vi "Highlight Text.vi"(7 "Values":refnum<vi>, 8 "error in (no error)":errorcluster, 9 "ASCII":refnum<vi>, 10 "Hex":refnum<vi>, 11 "queue data in":T1={"server ID"=refnum, "Buffer data"={"decimation"=0, "avg bandwidth"=0.0, "channels"=[], "byte order"=enum."little-endian", "buffer descriptor"={"buffer type"=enum."Engine", "plugin id"=0, "group id"=0, "transfer id"=0, "offset"=0, "length"=0}, "values channels"={"index"=0, "count"=0, "engine offset"=0}, "select start offset"=18446744073709551615, "select end offset"=0, "channel index"=-1}} {"Buffer data"."channels"."configuration"."string offset" format="%d bytes"; "Buffer data"."avg bandwidth" format="%.0g bytes"}) -> (0 "error out":errorcluster, 3 "queue data out":T1={"server ID"=refnum, "Buffer data"={"decimation"=0, "avg bandwidth"=0.0, "channels"=[], "byte order"=enum."little-endian", "buffer descriptor"={"buffer type"=enum."Engine", "plugin id"=0, "group id"=0, "transfer id"=0, "offset"=0, "length"=0}, "values channels"={"index"=0, "count"=0, "engine offset"=0}, "select start offset"=18446744073709551615, "select end offset"=0, "channel index"=-1}} {"Buffer data"."channels"."configuration"."string offset" format="%d bytes"; "Buffer data"."avg bandwidth" format="%.0g bytes"})   [LabVIEW 2017, in "DSF Core.lvlib"]
uses:
  DSF Core.lvlib
  Buffer Reader/Queue Data.ctl
  Buffer Reader/Buffer Data.ctl
  Classes/Configuration/Core/Transfer/Channel Configuration.ctl
  Typedefs/Core Channel Configuration.ctl
  Typedefs/DSF Data Type.ctl
  Typedefs/DSF Settings Info.ctl
  Typedefs/DSF Byte Order.ctl
  Classes/Thread/Data Server/DSF Buffer Subset Descriptor.ctl
  Typedefs/DSF Buffer Type.ctl
  Values Channels.ctl
  Classes/Configuration/Core/Channel/Channel Configuration.lvclass
  Classes/Configuration/Core/Transfer/Transfer Configuration.lvclass
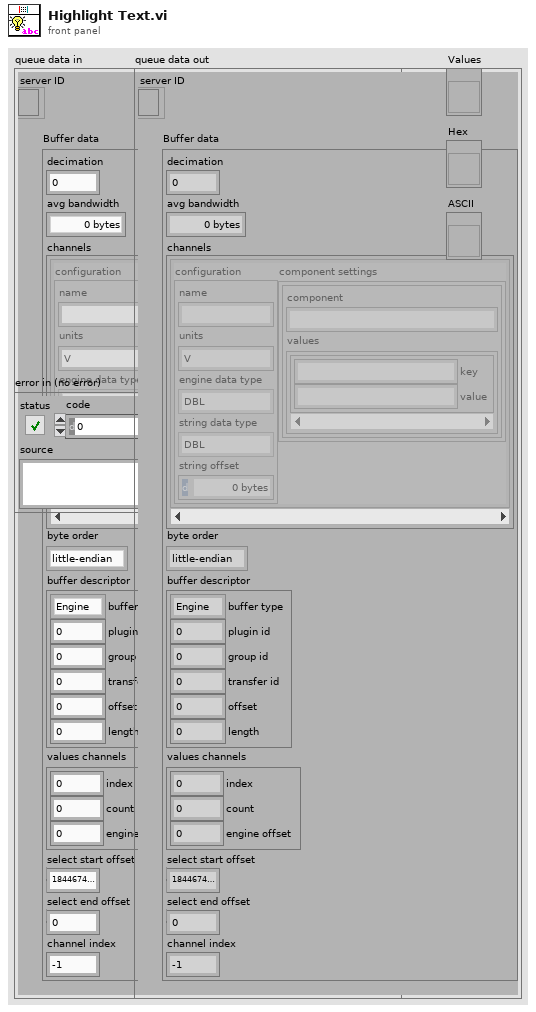
[diagram p1: front panel]
types:
  T1 = typedef "DSF Core.lvlib/Queue Data.ctl" = cluster{"server ID":refnum<k5>, "Buffer data":T2}
  T2 = typedef "DSF Core.lvlib/Buffer Data.ctl" = cluster{"decimation":u64, "avg bandwidth":dbl, "channels":T3[], "byte order":T7, "buffer descriptor":T8, "values channels":T10, "select start offset":u64, "select end offset":u64, "channel index":i32}
  T3 = typedef "DSF Core.lvlib/Transfer Configuration.lvclass/Channel Configuration.ctl" = cluster{"configuration":T4, "component settings":T6[]}
  T4 = typedef "DSF Core.lvlib/Channel Configuration.lvclass/Core Channel Configuration.ctl" = cluster{"name":string, "units":string, "engine data type":T5, "string data type":T5, "string offset":u64}
  T5 = typedef "DSF Core.lvlib/DSF Data Type.ctl" = enum8{"Bool", "SGL", "DBL", "I8", "I16", "I32", "I64", "U8", "U16", "U32", "U64"}
  T6 = typedef "DSF Core.lvlib/DSF Settings Info.ctl" = cluster{"component":string, "values":cluster{"key":string, "value":string}[]}
  T7 = typedef "DSF Core.lvlib/DSF Byte Order.ctl" = enum8{"big-endian", "little-endian"}
  T8 = typedef "DSF Core.lvlib/DSF Buffer Subset Descriptor.ctl" = cluster{"buffer type":T9, "plugin id":i32, "group id":i32, "transfer id":i32, "offset":u64, "length":i64}
  T9 = typedef "DSF Core.lvlib/DSF Buffer Type.ctl" = enum16{"Engine", "String"}
  T10 = typedef "DSF Core.lvlib/Values Channels.ctl" = cluster{"index":i32, "count":i32, "engine offset":u64}
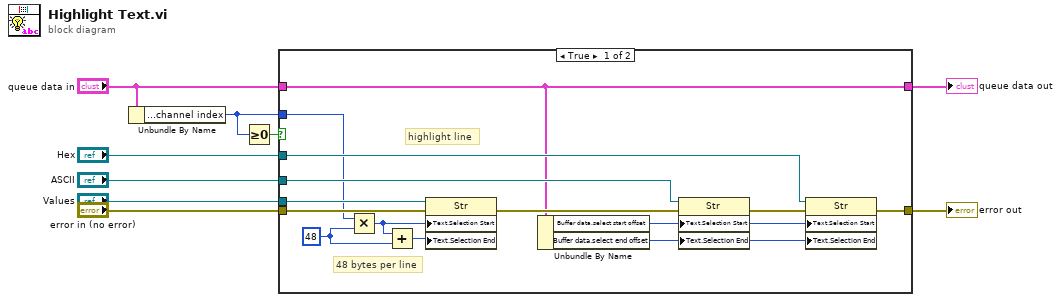
[diagram p0: block diagram]
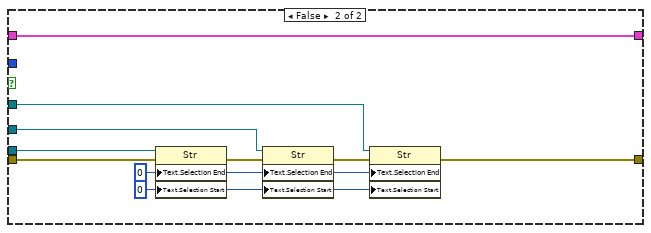
[diagram p2: hidden frame]
diagram:
  n1 = Unbundle By Name("queue data in") -> ("Buffer data.channel index"=w1:i32)
  n2 = Greater Or Equal To 0?(x=w1) -> (x >= 0?=w5:bool)
  n3 = case shown="True" w5 {
    tunnel: "ASCII" -> [w19 w28]
    tunnel: "Hex" -> [w14 w29]
    tunnel: [w12 w32] -> w9
    tunnel: "queue data in" -> [w11 w26]
    tunnel: [w11 w26] -> w8
    tunnel: "error in (no error)" -> [w22 w31]
    tunnel: "Values" -> [w20 w30]
    tunnel: w1 -> [w10 _]
    frame True {
      w17 = 48 ("y")
      # "highlight line"
      # "48 bytes per line"
      n4 = Multiply(x=w10, y=w17) -> (x*y=w15:i32)
      n5 = Add(x=w15, y=w17) -> (x+y=w16:i32)
      n6 = property class="Str"(reference=w20, error in=w22, "Text.Selection Start"=w15, "Text.Selection End"=w16) -> (error out=w18:errorcluster)  [unwired: 1 out]
      n7 = Unbundle By Name(w11) -> ("Buffer data.select start offset"=w13:u64, "Buffer data.select end offset"=w21:u64)
      n8 = property class="Str"(reference=w19, error in=w18, "Text.Selection Start"=w13, "Text.Selection End"=w21) -> (error out=w23:errorcluster)  [unwired: 1 out]
      n9 = property class="Str"(reference=w14, error in=w23, "Text.Selection Start"=w13, "Text.Selection End"=w21) -> (error out=w12:errorcluster)  [unwired: 1 out]
    }
    frame False {
      w24 = u32 0 ("Text.Selection:Start")
      w25 = u32 0 ("Text.Selection:End")
      n10 = property class="Str"(reference=w30, error in=w31, "Text.Selection End"=w25, "Text.Selection Start"=w24) -> (error out=w27:errorcluster)  [unwired: 1 out]
      n11 = property class="Str"(reference=w28, error in=w27, "Text.Selection End"=w25, "Text.Selection Start"=w24) -> (error out=w33:errorcluster)  [unwired: 1 out]
      n12 = property class="Str"(reference=w29, error in=w33, "Text.Selection End"=w25, "Text.Selection Start"=w24) -> (error out=w32:errorcluster)  [unwired: 1 out]
    }
  }
  "error out" <- w9
  "queue data out" <- w8
